vi "Gas_Status_panel.vi"(7 "Ch names":string[](array[string])) -> (1 "Trace Gas":string, 2 "Trace Hi-Tec Range":string, 4 "Channel 1":dbl format="%.2f", 6 "Channel 2":dbl format="%.2f", 8 "Signal FID Span":dbl format="%.2f", 10 "Gas Remaining":string[][](table), 12 "Carrier Gas 1":string, 13 "Carrier Gas 2":string, 14 "Carrier 1 Hi-Tec Range":string)   [LabVIEW 2010]
uses:
  Anemometry/Anemometry Sub Vis/Globals/Gas_management_global.vi
panel:
  out "Atmos Pres (mbars)":string
  out "Release temp (deg C)":dbl format="%.2f"
  # "Carrier Gas"
  # "Calibration Gas (ppm)"
  # "Trace Gas"
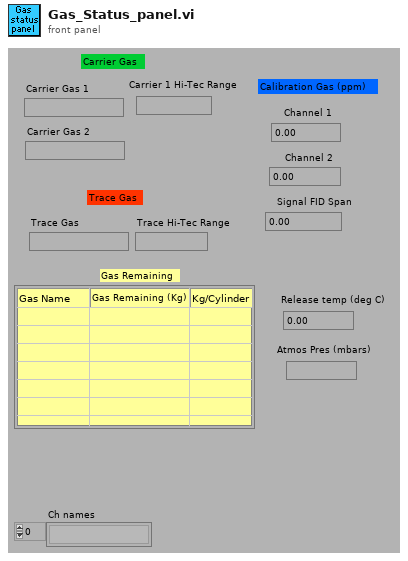
[diagram p1: front panel]
types:
  T1 = enum16{"Gas Remaining", "Trace Gas", "Carrier Gas", "Calibration Gas", "Atmospheric Pressure"}
  T2 = typedef "Ch_description_ADAM.ctl" = cluster{"Ch Name":string, "Type":T3, "Function":T4, "Ch State":T5, "Calibration type":T6, "A":dbl, "B":dbl, "C":dbl, "D":dbl, "Comments":string, "Address":T7, "String":string, "Duty":u16}
  T3 = typedef "Module_type_ADAM.ctl" = enum16{"4011", "4012", "4013", "4014", "4016", "4017", "4018", "4021", "4050", "4052", "4053", "4060", "4080", "5000", "5017", "5018", "5024", "5051", "5056", "5060", "6060", "Tracker", "WEST", "GILL", "JEM", "VICI", "Vaisala", "DRUCK", "Run VI Named:", "IR2100", "PPT", "Comparator", "VIRTUAL", "Hold Value", "Read A", "Read Ch", "Coded", "Client Info", "Web Client", "X10", "Test"}
  T4 = typedef "Function_ADAM.ctl" = enum16{"Analogue Input", "Digital Input", "Event counter", "Event rate", "Analogue Output", "Digital Output", "Relay Output"}
  T5 = typedef "Channel_State.ctl" = enum16{"On", "Off", "Always On", "Always Off"}
  T6 = typedef "Calib_type_ADAM.ctl" = enum16{"Raw", "Bx + A", "Cx^2 + Bx + A", "Dx^3 + Cx^2 + Bx + A", "In Band", "Hi-Tec Q", "Hi-Tec M_dot", "Text"}
  T7 = typedef "Address.ctl" = cluster{"Main":i32, "Ch.":i32, "Sub":i32, "Port Name":string}
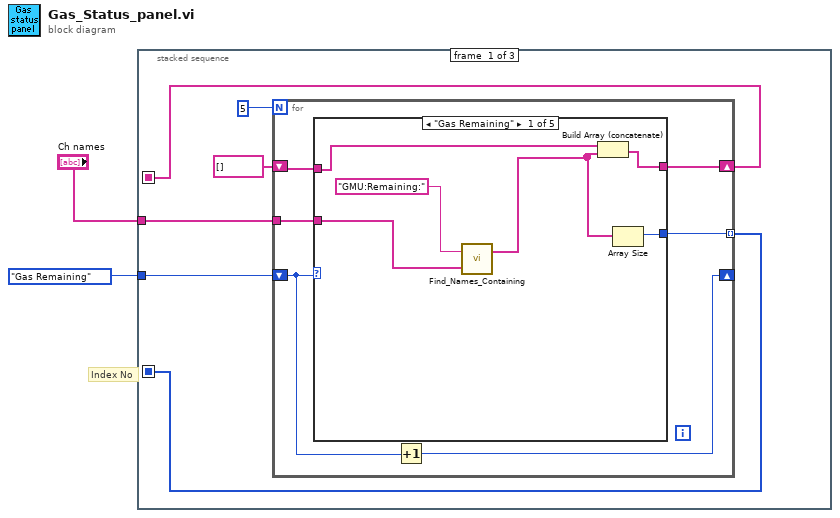
[diagram p0: block diagram]
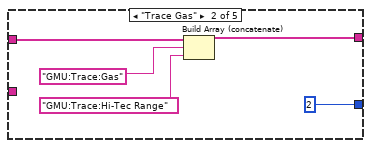
[diagram p2: hidden frame]
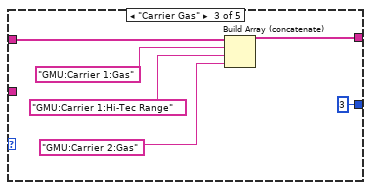
[diagram p3: hidden frame]
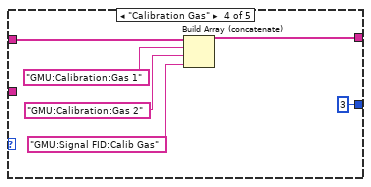
[diagram p4: hidden frame]
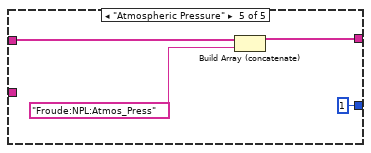
[diagram p5: hidden frame]
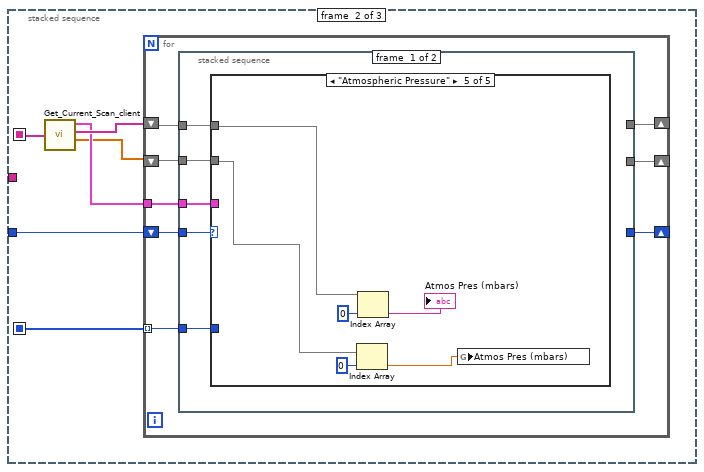
[diagram p6: hidden frame]
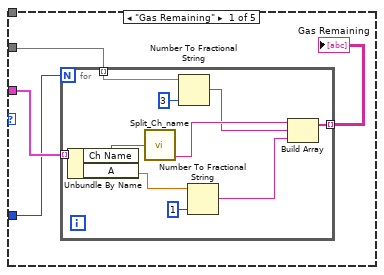
[diagram p7: hidden frame]
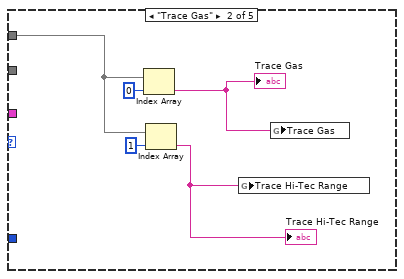
[diagram p8: hidden frame]
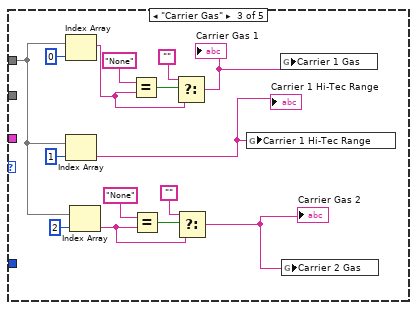
[diagram p9: hidden frame]
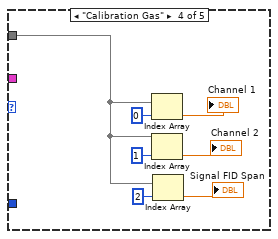
[diagram p10: hidden frame]
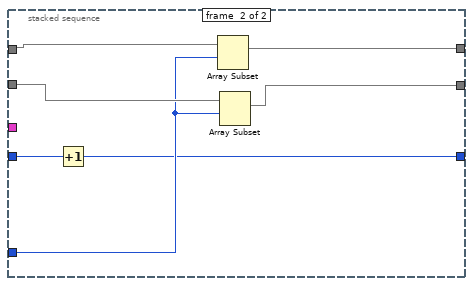
[diagram p11: hidden frame]
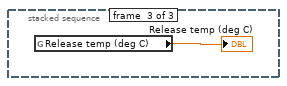
[diagram p12: hidden frame]
diagram:
  # "Index No"
  n1 = stacked-sequence {
    seq-local: [w6 _ _] -> [_ w46 _]
    seq-local: [w4 _ _] -> [_ w43 _]
    tunnel: T1."Gas Remaining" -> [w8 w47 _]
    tunnel: "Ch names" -> [w5 _ _]
    frame #0 {
      n2 = for {
        N: 5 -> [_]
        shift-right: [w13] -> _
        shift-left: w8 -> [w14]
        shift-right: [w11] -> w6
        shift-left: string[] [] -> [w12]
        tunnel: w5 -> [w10]
        tunnel: [w9] -> w4 mode=indexing
        n3 = case shown="\"Gas Remaining\"" w14 {
          tunnel: w12 -> [w19 w25 w31 w37 w41]
          tunnel: [w18 w24 w30 w36 w40] -> w11
          tunnel: w10 -> [w20 _ _ _ _]
          tunnel: [w16 2 3 3 1] -> w9
          frame "Gas Remaining" {
            n4 = call "Find_Names_Containing.vi"("Ch names"=w20, "String to match"="GMU:Remaining:") -> ("Matched Names"=w17:string[])  [unwired: 1 out]
            n5 = Build Array (concatenate)(w19, w17) -> (w18:string[])
            n6 = Array Size(array=w17) -> (size(s)=w16:i32)
          }
          frame "Trace Gas" {
            n7 = Build Array (concatenate)(w25, "GMU:Trace:Gas", "GMU:Trace:Hi-Tec Range") -> (w24:string[])
          }
          frame "Carrier Gas" {
            n8 = Build Array (concatenate)(w31, "GMU:Carrier 1:Gas", "GMU:Carrier 1:Hi-Tec Range", "GMU:Carrier 2:Gas") -> (w30:string[])
          }
          frame "Calibration Gas" {
            n9 = Build Array (concatenate)(w37, "GMU:Calibration:Gas 1", "GMU:Calibration:Gas 2", "GMU:Signal FID:Calib Gas") -> (w36:string[])
          }
          frame "Atmospheric Pressure" {
            n10 = Build Array (concatenate)(w41, "Froude:NPL:Atmos_Press") -> (w40:string[])
          }
        }
        n11 = Increment(x=w14) -> (x+1=w13:T1)
      }
    }
    frame #1 {
      n12 = call "Get_Current_Scan_client.vi"("ADAM Ch Names"=w46) -> ("Ch Description Array"=w44:T2[], "String values"=w45:string[], "Numerical Values"=w42:dbl[])  [unwired: 1 out]
      n13 = for {
        shift-right: [w48] -> _
        shift-left: w47 -> [w53]
        shift-right: [w54] -> _
        shift-left: w45 -> [w55]
        tunnel: w44 -> [w52]
        tunnel: w43 -> [w51] mode=indexing
        shift-right: [w49] -> _
        shift-left: w42 -> [w50]
        n14 = stacked-sequence {
          tunnel: w55 -> [w60 w114]
          tunnel: [_ w111] -> w54
          tunnel: w53 -> [w59 w109]
          tunnel: w52 -> [w58 _]
          tunnel: w51 -> [w57 w112]
          tunnel: w50 -> [w56 w113]
          tunnel: [_ w110] -> w49
          tunnel: [_ w108] -> w48
          frame #0 {
            n15 = case shown="\"Atmospheric Pressure\"" w59 {
              tunnel: w60 -> [_ w75 w90 _ w103]
              tunnel: w58 -> [w64 _ _ _ _]
              tunnel: w57 -> [w62 _ _ _ _]
              tunnel: w56 -> [w61 _ _ w95 w102]
              frame "Gas Remaining" {
                n16 = for {
                  N: w62 -> [_]
                  tunnel: w64 -> [w74] mode=indexing
                  tunnel: [w68] -> w63 mode=indexing
                  tunnel: w61 -> [w66] mode=indexing
                  n17 = Unbundle By Name(w74) -> ("Ch Name"=w73:string, "A"=w71:dbl)
                  n18 = call "Split_Ch_name.vi"("Ch name"=w73) -> ("Low level"=w70:string)  [unwired: 2 out]
                  n19 = Number To Fractional String(number=w66, precision (6)=i16 3) -> (F-format string=w65:string)  [unwired: 2 out]
                  n20 = Number To Fractional String(number=w71, precision (6)=i16 1) -> (F-format string=w69:string)  [unwired: 2 out]
                  n21 = Build Array(w70, w65, w69) -> (w68:string[])
                }
                "Gas Remaining" <- w63
              }
              frame "Trace Gas" {
                n22 = Index Array(array=w75, index=0) -> (element=w77:string)
                "Trace Gas" <- w77
                n23 = Index Array(array=w75, index=1) -> (element=w76:string)
                "Trace Hi-Tec Range" <- w76
                n24 = global write "Gas_management_global.vi" "Trace Hi-Tec Range"(w76) -> ()
                n25 = global write "Gas_management_global.vi" "Trace Gas"(w77) -> ()
              }
              frame "Carrier Gas" {
                n26 = Index Array(array=w90, index=0) -> (element=w81:string)
                n27 = Index Array(array=w90, index=1) -> (element=w92:string)
                "Carrier 1 Hi-Tec Range" <- w92
                n28 = Index Array(array=w90, index=2) -> (element=w87:string)
                n29 = Equal?(x="None" ("y"), y=w81) -> (x = y?=w82:bool)
                n30 = Equal?(x="None" ("y"), y=w87) -> (x = y?=w89:bool)
                n31 = Select(t="", s=w82, f=w81) -> (s? t:f=w80:string)
                "Carrier Gas 1" <- w80
                n32 = Select(t="", s=w89, f=w87) -> (s? t:f=w85:string)
                "Carrier Gas 2" <- w85
                n33 = global write "Gas_management_global.vi" "Carrier 1 Hi-Tec Range"(w92) -> ()
                n34 = global write "Gas_management_global.vi" "Carrier 1 Gas"(w80) -> ()
                n35 = global write "Gas_management_global.vi" "Carrier 2 Gas"(w85) -> ()
              }
              frame "Calibration Gas" {
                n36 = Index Array(array=w95, index=0) -> (element=→"Channel 1":dbl)
                n37 = Index Array(array=w95, index=1) -> (element=→"Channel 2":dbl)
                n38 = Index Array(array=w95, index=2) -> (element=→"Signal FID Span":dbl)
              }
              frame "Atmospheric Pressure" {
                n39 = Index Array(array=w102, index=0) -> (element=w104:dbl)
                n40 = Index Array(array=w103, index=0) -> (element=→"Atmos Pres (mbars)":string)
                n41 = global write "Gas_management_global.vi" "Atmos Pres (mbars)"(w104) -> ()
              }
            }
          }
          frame #1 {
            n42 = Increment(x=w109) -> (x+1=w108:T1)
            n43 = Array Subset(array=w114, index=w112) -> (w111:string[])  [unwired: 1 in]
            n44 = Array Subset(array=w113, index=w112) -> (w110:dbl[])  [unwired: 1 in]
          }
        }
      }
    }
    frame #2 {
      n45 = global read "Gas_management_global.vi" "Release temp (deg C)"() -> (→"Release temp (deg C)":dbl)
    }
  }
